vi "temp.vi"() -> ()   [LabVIEW 2013]
uses:
  magnet polar field.ctl
  config.vi
panel:
  in  "magnet polar":T1
  in  "User Defined ramp rate":dbl=0.005 format="%#_13g"
  out "error out":T2
  in  "error in":T2
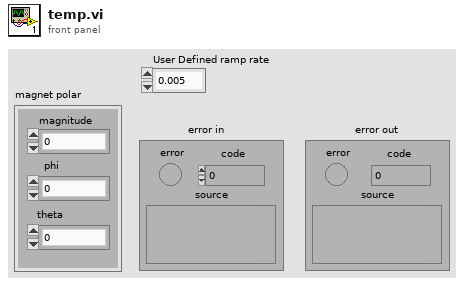
[diagram p1: front panel]
types:
  T1 = typedef "magnet polar field.ctl" = cluster{"magnitude":dbl, "phi":dbl, "theta":dbl}
  T2 = cluster{"error":bool, "code":i32, "source":string}
  T3 = cluster{"GPIB address":i16, "GPIB bus":i16, "connection ID":refnum<k5>, "IP":string, "Active Comm Interface":u16, "Serial Port":refnum<visa-resource-name>, "Programmer Type":u16}
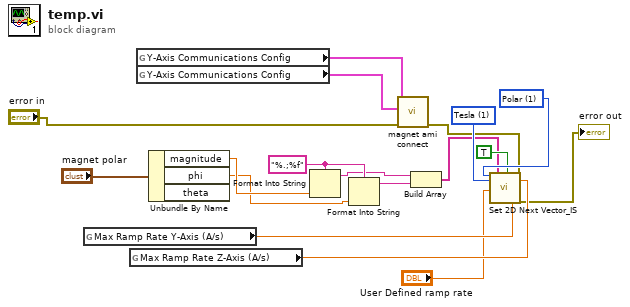
[diagram p0: block diagram]
diagram:
  w6 = "%.;%f" ("format string")
  w14 = u16 1 items=["Cartesian", "Polar"] ("Coordinate System")
  w15 = u16 1 items=["kG", "Tesla"] ("Magnetic Field Units")
  n1 = global read "config.vi" "Max Ramp Rate Y-Axis (A/s)"() -> (w16:dbl)
  n2 = global read "config.vi" "Max Ramp Rate Z-Axis (A/s)"() -> (w13:dbl)
  n3 = global read "config.vi" "Y-Axis Communications Config"() -> (w18:T3)
  n4 = global read "config.vi" "Y-Axis Communications Config"() -> (w17:T3)
  n5 = Unbundle By Name("magnet polar") -> ("magnitude"=w2:dbl, "phi"=w1:dbl)  [unwired: 1 out]
  n6 = Format Into String(format string=w6, w2) -> (resulting string=w5:string)  [unwired: 2 in, 1 out]
  n7 = Format Into String(format string=w6, w1) -> (resulting string=w4:string)  [unwired: 2 in, 1 out]
  n8 = call "magnet ami connect.vi"("error in (no error)"="error in", "Z-Axis Communications Config"=w17, "Y-Axis Communications Config"=w18) -> ("error out"=w12:errorcluster)  [unwired: 6 in, 2 out]
  n9 = Build Array(w5, w4) -> (w3:string[])
  n10 = call "Set 2D Next Vector_IS.vi"("Coordinate System"=w14, "Magnetic Field Units"=w15, 3:"User defined Ramp Rate (T/min)"="User Defined ramp rate", "Input Vector"=w3, 10:"User defined Ramp Rate (T/min)"=TRUE ("User defined Ramp Rate (T/min)"), "Max Ramp Rate - Y Axis (A/s)"=w16, "error in"=w12, "Max Ramp Rate - Z Axis (A/s)"=w13) -> ("error out"=→"error out":T2)  [unwired: 6 in, 5 out]
